vi "Gyro Steer.vi"(9 "Turn Speed":dbl, 10 "Target Angle":dbl, 11 "Changed?":bool) -> (1 "In Range?":bool, 3 "X out":dbl)   [LabVIEW 2016]
uses:
  Robot Global Data.vi
  <vilib>/addons/control/pid/pid.llb/PID (DBL).vi
  <vilib>/addons/control/pid/NI_PID_pid.lvlib
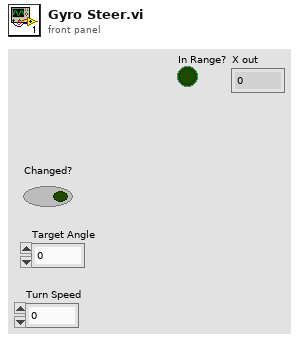
[diagram p1: front panel]
types:
  T1 = typedef "Dashboard Control Data.ctl" = cluster{"Intake Presets":T2, "Drivetrain Presets":T3}
  T2 = typedef "Intake Presets.ctl" = cluster{"Intake Power":dbl, "Outtake Power":dbl}
  T3 = typedef "Drivetrain Presets.ctl" = cluster{"Steer PID output":cluster{"output high":dbl, "output low":dbl}, " Steer PID gains":cluster{"proportional gain (Kc)":dbl, "integral time (Ti, min)":dbl, "derivative time (Td, min)":dbl}, "Gyro Tolerance":dbl}
  T4 = cluster{"proportional gain (Kc)":dbl, "integral time (Ti, min)":dbl, "derivative time (Td, min)":dbl}
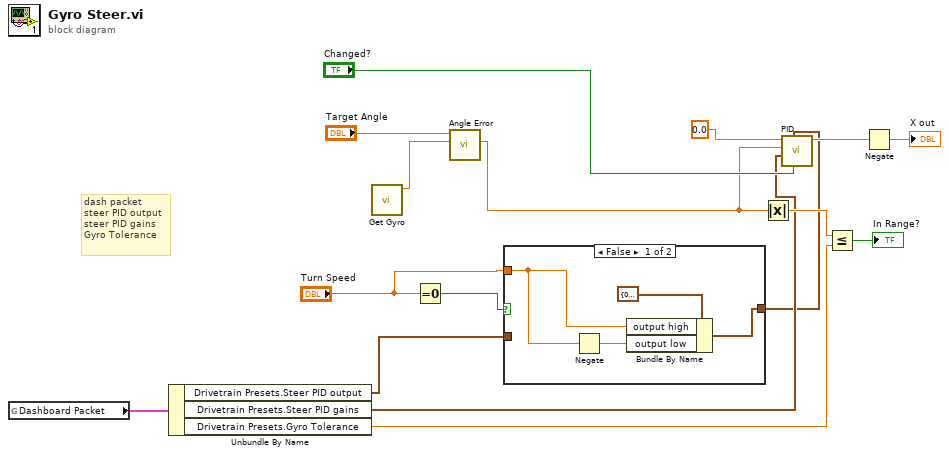
[diagram p0: block diagram]
diagram:
  # "dash packet \nsteer PID output\nsteer PID gains\nGyro Tolerance"
  n1 = global read "Robot Global Data.vi" "Dashboard Packet"() -> (w5:T1)
  n2 = Unbundle By Name(w5) -> ("Drivetrain Presets.Steer PID output"=w3:cluster{"output high":dbl, "output low":dbl}, "Drivetrain Presets.Steer PID gains"=w4:T4, "Drivetrain Presets.Gyro Tolerance"=w1:dbl)
  n3 = call "Get Gyro.vi"() -> ("Angle"=w7:dbl)  [unwired: 11 in]
  n4 = Equal To 0?(x="Turn Speed") -> (x = 0?=w16:bool)
  n5 = call "Angle Error.vi"("Angle"=w7, "Target Angle"="Target Angle") -> ("Error"=w6:dbl)  [unwired: 9 in]
  n6 = case shown="False" w16 {
    tunnel: "Turn Speed" -> [w17 _]
    tunnel: w3 -> [_ w21]
    tunnel: [w19 w21] -> w2
    frame False {
      n7 = Negate(x=w17) -> (-x=w18:dbl)
      n8 = Bundle By Name(cluster=cluster{"output high":dbl, "output low":dbl} {"output high"=0.0, "output low"=0.0} ("Steer PID output Range"), "output high"=w17, "output low"=w18) -> (w19:cluster{"output high":dbl, "output low":dbl})
    }
    frame True {
    }
  }
  n9 = Absolute Value(x=w6) -> (abs(x)=w12:dbl)
  n10 = call-poly <vilib>:"PID.vi"("reinitialize? (F)"="Changed?", "output range"=w2, "PID gains"=w4, "process variable"=w6, "setpoint"=0.0) -> ("output"=w10:dbl)  [unwired: 5 in, 1 out]
  n11 = Less Or Equal?(x=w12, y=w1) -> (x <= y?=→"In Range?":bool)
  n12 = Negate(x=w10) -> (-x=→"X out":dbl)
